vi "Configure Current Low Limit.vi"(0 "VISA resource name":refnum<visa-resource-name>, 5 "Current Low Limit (0 A)":dbl min=0.0 max=36.8 format="%.3f", 11 "error in (no error)":errorcluster) -> (4 "VISA resource name out":refnum<visa-resource-name>, 15 "error out":errorcluster)   [LabVIEW 2014, in "eec 6700.lvlib"]
doc: "Sets the <B>Current Low Limit</B> in the active step of the power source instrument.\n\n<B>Range</B> : 0.000~33.6 A\n\nModel | Voltage Range | RMS Current\n------------------------------------------------\n 6705 | (0-150 V) - Auto | 0.00 - 4.20 A\n 6705 | (0-300 V) - High | 0.00 - 2.10 A\n---------------------------------------------\n 6710 | (0-150 V) - Auto | 0.00 - 8.40 A\n 6710 | (0-300 V) - High | 0.00 - 4.20 A\n--------------------------------------\n 6720 | (0-150 V) - Auto | 0.00 - 16.80 A\n 6720 | (0-300 V) - High | 0.00 - 8.40 A\n--------------------------------------\n 6730 | (0-150 V) - Auto | 0.00 - 25.20 A\n 6730 | (0-300 V) - High | 0.00 - 12.60 A\n--------------------------------------\n 6740 | (0-150 V) - Auto | 0.00 - 33.60 A\n 6740 | (0-300 V) - High | 0.00 - 16.80 A\n\nThe current Low-Limit setting configures a minimum current threshold or floor level. If a minimum current level is not reached a test failure will occur. This insures a load is attached to the power source and there is a minimum current present."
uses:
  <instrlib>/eec 6700/eec 6700.lvlib
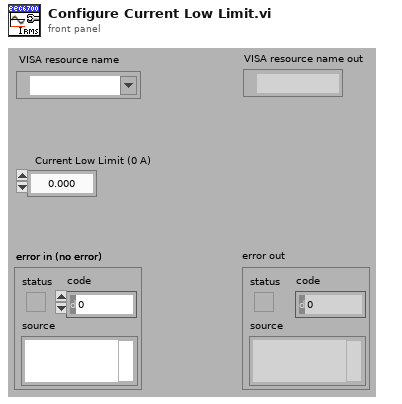
[diagram p1: front panel]
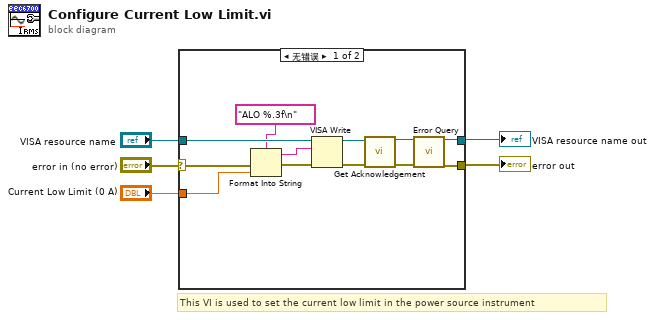
[diagram p0: block diagram]
diagram:
  # "This VI is used to set the current low limit in the power source instrument"
  n1 = case shown="无错误" "error in (no error)" {
    selector: "error in (no error)" -> [w11 w19]
    tunnel: "VISA resource name" -> [w17 w18]
    tunnel: [w13 w18] -> w4
    tunnel: [w12 w19] -> w3
    tunnel: "Current Low Limit (0 A)" -> [w16 _]
    frame No Error {
      n2 = Format Into String(format string="ALO %.3f\n" ("Command"), error in=w11, w16) -> (resulting string=w15:string, error out=w10:errorcluster)  [unwired: 1 in]
      n3 = VISA Write(VISA resource name=w17, write buffer=w15, error in (no error)=w10) -> (VISA resource name out=w7:refnum<visa-resource-name>, error out=w9:errorcluster)  [unwired: 1 out]
      n4 = call <instrlib>:"Get Acknowledgement.vi"("VISA resource name"=w7, "error in (no error)"=w9) -> ("VISA resource name out"=w6:refnum<visa-resource-name>, "error out"=w8:errorcluster)  [unwired: 12 in]
      n5 = call <instrlib>:"Error Query.vi"("VISA resource name"=w6, "error in (no error)"=w8) -> ("VISA resource name out"=w13:refnum<visa-resource-name>, "error out"=w12:errorcluster)  [unwired: 10 in, 2 out]
    }
    frame Error {
    }
  }
  "error out" <- w3
  "VISA resource name out" <- w4
